vi "Save Configuration Coins.vi"(8 "error in (no error)":errorcluster, 11 "Coins":cluster{"Bolean text":string, "Value":i32}[](array[cluster])) -> (0 "error out":errorcluster)   [LabVIEW 2019, in "Monedas.lvlib"]
uses:
  Monedas.lvlib
  <vilib>/Utility/xml.llb/Write to XML File(string).vi
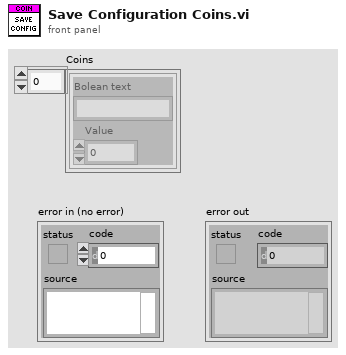
[diagram p1: front panel]
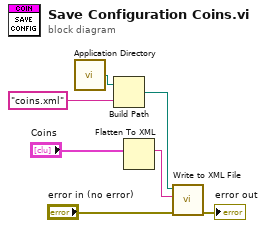
[diagram p0: block diagram]
diagram:
  n1 = call <vilib>:"Application Directory.vi"() -> ("Application Directory"=w7:path)
  n2 = Build Path(base path=w7, name or relative path="coins.xml") -> (appended path=w4:path)
  n3 = Flatten To XML(anything="Coins") -> (xml string=w3:string)
  n4 = call-poly <vilib>:"Write to XML File.vi"("error in (no error)"="error in (no error)", "XML Input"=w3, "XML File Path"=w4) -> ("error out"=→"error out":errorcluster)  [unwired: 6 in, 2 out]
